vi "Find SPINE Direction (SubVI).vi"(10 "Point 2":u64, 11 "Point 1":u64) -> (3 "Reverse?":bool)   [LabVIEW 2015]
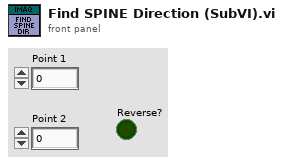
[diagram p1: front panel]
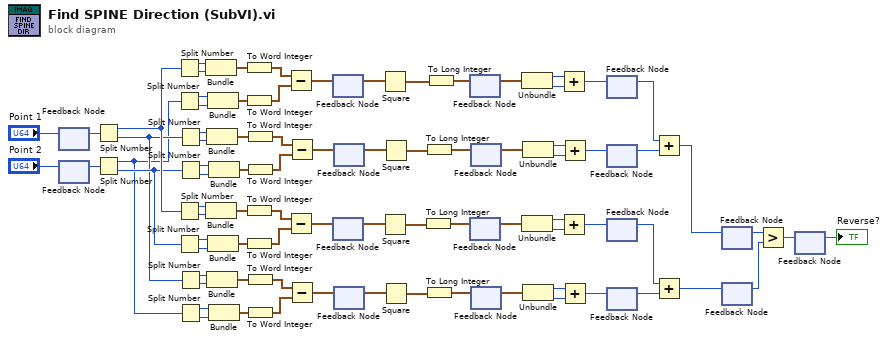
[diagram p0: block diagram]
diagram:
  n1 = feedback-in #1("Point 1") -> ()
  n2 = feedback #1() -> (w76:u64)  [unwired: 1 in]
  n3 = feedback-in #2("Point 2") -> ()
  n4 = feedback #2() -> (w75:u64)  [unwired: 1 in]
  n5 = Split Number(x=w76) -> (hi(x)=w23:u32, lo(x)=w21:u32)
  n6 = Split Number(x=w75) -> (hi(x)=w20:u32, lo(x)=w22:u32)
  n7 = Split Number(x=w23) -> (hi(x)=w73:u16, lo(x)=w72:u16)
  n8 = Split Number(x=w20) -> (hi(x)=w70:u16, lo(x)=w69:u16)
  n9 = Split Number(x=w23) -> (hi(x)=w24:u16, lo(x)=w18:u16)
  n10 = Split Number(x=w22) -> (hi(x)=w26:u16, lo(x)=w27:u16)
  n11 = Split Number(x=w21) -> (hi(x)=w50:u16, lo(x)=w51:u16)
  n12 = Split Number(x=w22) -> (hi(x)=w53:u16, lo(x)=w54:u16)
  n13 = Split Number(x=w21) -> (hi(x)=w45:u16, lo(x)=w17:u16)
  n14 = Split Number(x=w20) -> (hi(x)=w43:u16, lo(x)=w42:u16)
  n15 = Bundle(w73, w72) -> (w68:cluster{u16, u16})  [unwired: 1 in]
  n16 = Bundle(w24, w18) -> (w28:cluster{u16, u16})  [unwired: 1 in]
  n17 = Bundle(w50, w51) -> (w55:cluster{u16, u16})  [unwired: 1 in]
  n18 = Bundle(w45, w17) -> (w41:cluster{u16, u16})  [unwired: 1 in]
  n19 = Bundle(w70, w69) -> (w67:cluster{u16, u16})  [unwired: 1 in]
  n20 = Bundle(w26, w27) -> (w29:cluster{u16, u16})  [unwired: 1 in]
  n21 = Bundle(w53, w54) -> (w56:cluster{u16, u16})  [unwired: 1 in]
  n22 = Bundle(w43, w42) -> (w40:cluster{u16, u16})  [unwired: 1 in]
  n23 = To Word Integer(number=w68) -> (16bit integer=w66:cluster{i16, i16})
  n24 = To Word Integer(number=w67) -> (16bit integer=w65:cluster{i16, i16})
  n25 = To Word Integer(number=w28) -> (16bit integer=w30:cluster{i16, i16})
  n26 = To Word Integer(number=w29) -> (16bit integer=w31:cluster{i16, i16})
  n27 = To Word Integer(number=w55) -> (16bit integer=w57:cluster{i16, i16})
  n28 = To Word Integer(number=w56) -> (16bit integer=w58:cluster{i16, i16})
  n29 = To Word Integer(number=w41) -> (16bit integer=w39:cluster{i16, i16})
  n30 = To Word Integer(number=w40) -> (16bit integer=w38:cluster{i16, i16})
  n31 = Subtract(x=w66, y=w65) -> (x-y=w71:cluster{i16, i16})
  n32 = Subtract(x=w30, y=w31) -> (x-y=w25:cluster{i16, i16})
  n33 = Subtract(x=w57, y=w58) -> (x-y=w52:cluster{i16, i16})
  n34 = Subtract(x=w39, y=w38) -> (x-y=w44:cluster{i16, i16})
  n35 = feedback-in #3(w71) -> ()
  n36 = feedback #3() -> (w8:cluster{i16, i16})  [unwired: 1 in]
  n37 = feedback-in #4(w25) -> ()
  n38 = feedback #4() -> (w6:cluster{i16, i16})  [unwired: 1 in]
  n39 = feedback-in #5(w52) -> ()
  n40 = feedback #5() -> (w7:cluster{i16, i16})  [unwired: 1 in]
  n41 = feedback-in #6(w44) -> ()
  n42 = feedback #6() -> (w5:cluster{i16, i16})  [unwired: 1 in]
  n43 = Square(x=w8) -> (x^2=w64:cluster{i16, i16})
  n44 = Square(x=w6) -> (x^2=w32:cluster{i16, i16})
  n45 = Square(x=w7) -> (x^2=w59:cluster{i16, i16})
  n46 = Square(x=w5) -> (x^2=w37:cluster{i16, i16})
  n47 = To Long Integer(number=w32) -> (32bit integer=w2:cluster{i32, i32})
  n48 = To Long Integer(number=w59) -> (32bit integer=w3:cluster{i32, i32})
  n49 = To Long Integer(number=w37) -> (32bit integer=w1:cluster{i32, i32})
  n50 = To Long Integer(number=w64) -> (32bit integer=w4:cluster{i32, i32})
  n51 = feedback-in #7(w4) -> ()
  n52 = feedback #7() -> (w12:cluster{i32, i32})  [unwired: 1 in]
  n53 = feedback-in #8(w2) -> ()
  n54 = feedback #8() -> (w10:cluster{i32, i32})  [unwired: 1 in]
  n55 = feedback-in #9(w3) -> ()
  n56 = feedback #9() -> (w11:cluster{i32, i32})  [unwired: 1 in]
  n57 = feedback-in #10(w1) -> ()
  n58 = feedback #10() -> (w9:cluster{i32, i32})  [unwired: 1 in]
  n59 = Unbundle(w12) -> (w63:i32, w62:i32)
  n60 = Unbundle(w10) -> (w33:i32, w34:i32)
  n61 = Unbundle(w11) -> (w60:i32, w61:i32)
  n62 = Unbundle(w9) -> (w36:i32, w35:i32)
  n63 = Add(x=w63, y=w62) -> (x+y=w49:i32)
  n64 = Add(x=w33, y=w34) -> (x+y=w46:i32)
  n65 = Add(x=w60, y=w61) -> (x+y=w48:i32)
  n66 = Add(x=w36, y=w35) -> (x+y=w47:i32)
  n67 = feedback-in #11(w49) -> ()
  n68 = feedback #11() -> (w16:i32)  [unwired: 1 in]
  n69 = feedback-in #12(w48) -> ()
  n70 = feedback #12() -> (w15:i32)  [unwired: 1 in]
  n71 = feedback-in #13(w46) -> ()
  n72 = feedback #13() -> (w14:i32)  [unwired: 1 in]
  n73 = feedback-in #14(w47) -> ()
  n74 = feedback #14() -> (w13:i32)  [unwired: 1 in]
  n75 = Add(x=w16, y=w15) -> (x+y=w80:i32)
  n76 = Add(x=w14, y=w13) -> (x+y=w19:i32)
  n77 = feedback-in #15(w80) -> ()
  n78 = feedback #15() -> (w78:i32)  [unwired: 1 in]
  n79 = feedback-in #16(w19) -> ()
  n80 = feedback #16() -> (w77:i32)  [unwired: 1 in]
  n81 = Greater?(x=w78, y=w77) -> (0:w79:bool)
  n82 = feedback-in #17(w79) -> ()
  n83 = feedback #17() -> (→"Reverse?":bool)  [unwired: 1 in]
